vi "Facade.vi"(0 "Data In":T4, 2 "Display State In":T2, 3 "Container State":T3) -> (6 "Data Out":T4, 7 "Display State Out":T2, 8 "Action":T1)   [LabVIEW 2020, in "TTLControlledDevice.xctl"]
uses:
  TTLControlledDevice.xctl
  Data.ctl
  Device Classes/Base Class/TTLControlledDevice.lvclass
  D:/Development/epl-vi-lib/Koop/KObject Class/KObject.lvclass
  <vilib>/_xctls/Container State.ctl
  State.ctl
  <vilib>/_xctls/Action.ctl
  epl-vi-lib/Utility VIs/Controls/KMultilevel Ring/KMultilevel Ring.xctl
  TTLWaterDelivery XControl/TTLWaterDelivery.xctl
  Device Classes/WaterDelivery Class/TTLWaterDelivery.lvclass
  D:/Development/epl-tosca/LV Source/TTL VIs/Device Classes/Base Class/TTLControlledDevice.lvclass
  Device Classes/Base Class/TTLControlledDevice.lvclass/TTLControlledDevice.ctl
  Device Classes/Base Class/Read Line.vi
  Device Classes/Base Class/Read Name.vi
  Device Classes/Base Class/Write Line.vi
  Device Classes/Base Class/Write Name.vi
  <vilib>/DAQmx/write.llb/DAQmx Write (Digital Bool 1Line 1Point).vi
  <vilib>/DAQmx/create/channels.llb/DAQmx Create Channel (DO-Digital Output).vi
  <vilib>/DAQmx/miscellaneous.llb/DAQmx Fill In Error Info.vi
  <vilib>/_xctls/XControlSupport.lvlib
panel:
  in  "Name":string
  out "water cal":bool
  in  "show class":i32
  in  "Class specific":enum32{"Page 1", "Page 2"}(tab)
  in  "Water":refnum<class "TTLWaterDelivery.lvclass">(xcontrol)
  in  "Line":string(xcontrol)
  in  "Test":bool
  out "Icon":picture
  in  "Type":u16(ring)
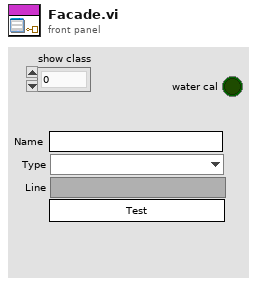
[diagram p1: front panel]
types:
  T1 = typedef "XControlSupport.lvlib/Action.ctl" = cluster{"Data Changed?":bool, "State Changed?":bool, "Action Name":string}
  T2 = typedef "TTLControlledDevice.xctl/State.ctl" = cluster{"Class Map":string[][], "Lines":string[]}
  T3 = typedef "XControlSupport.lvlib/Container State.ctl" = cluster{"Indicator?":bool, "Run Mode?":bool, " Refnum":refnum<vi>}
  T4 = typedef "TTLControlledDevice.xctl/Data.ctl" = refnum<class "TTLControlledDevice.lvclass">
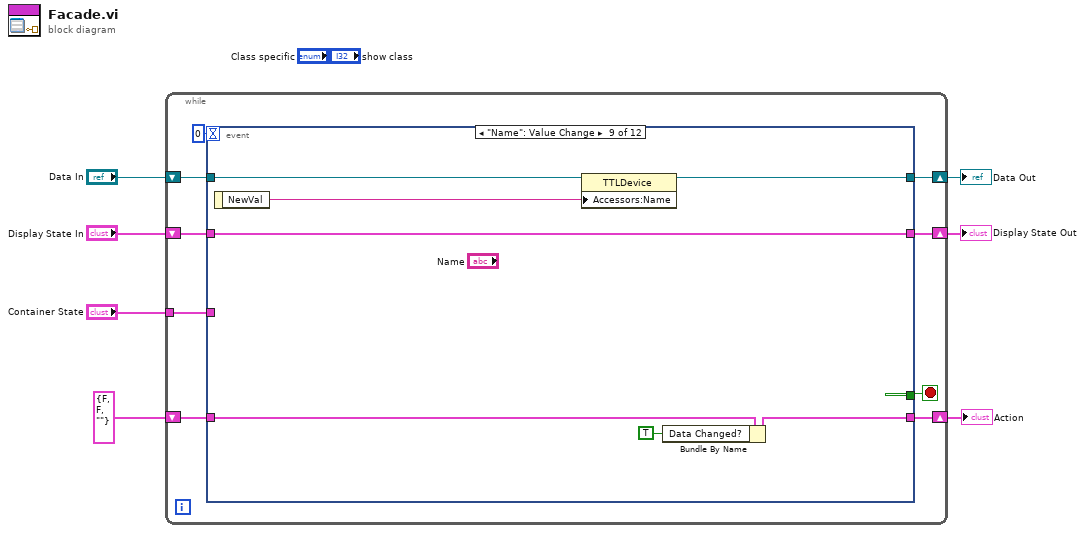
[diagram p0: block diagram]
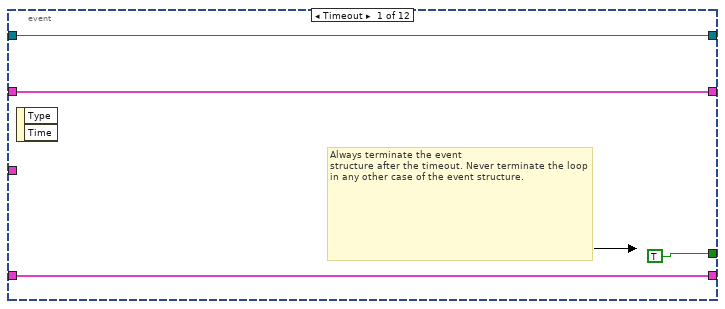
[diagram p2: hidden frame]
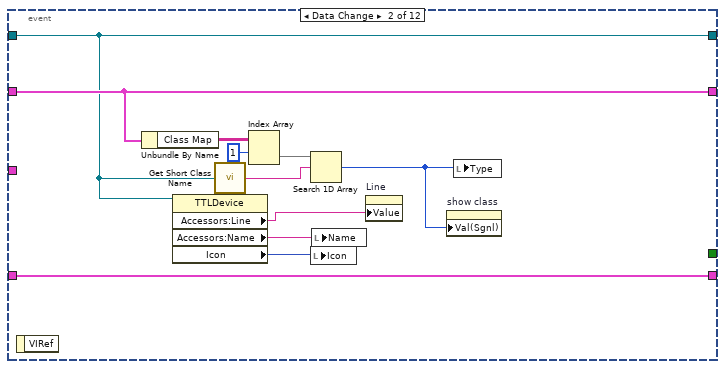
[diagram p3: hidden frame]
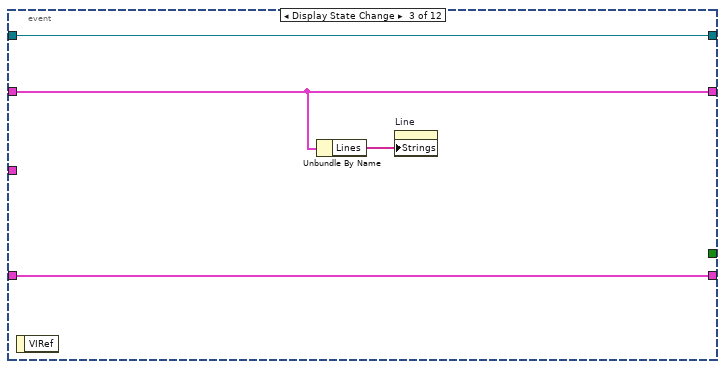
[diagram p4: hidden frame]
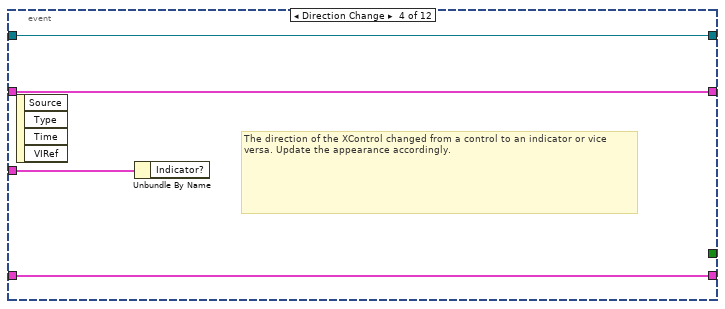
[diagram p5: hidden frame]
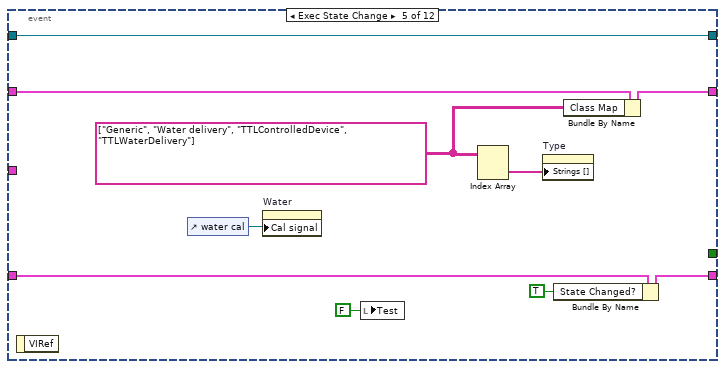
[diagram p6: hidden frame]
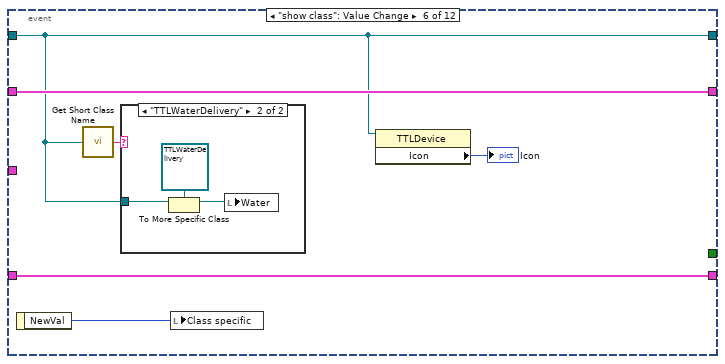
[diagram p7: hidden frame]
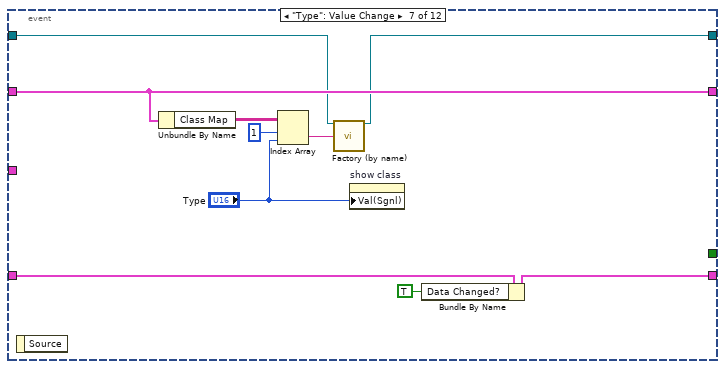
[diagram p9: hidden frame]
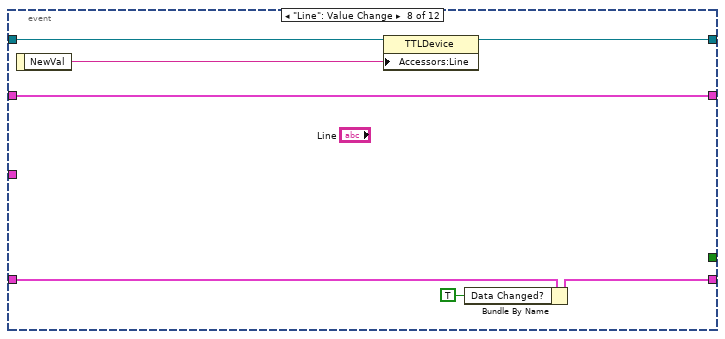
[diagram p10: hidden frame]
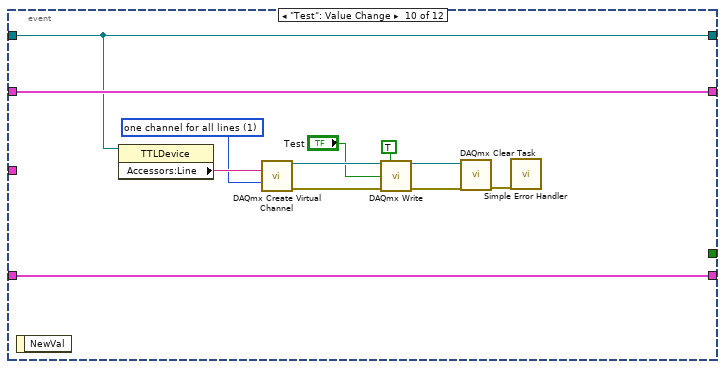
[diagram p11: hidden frame]
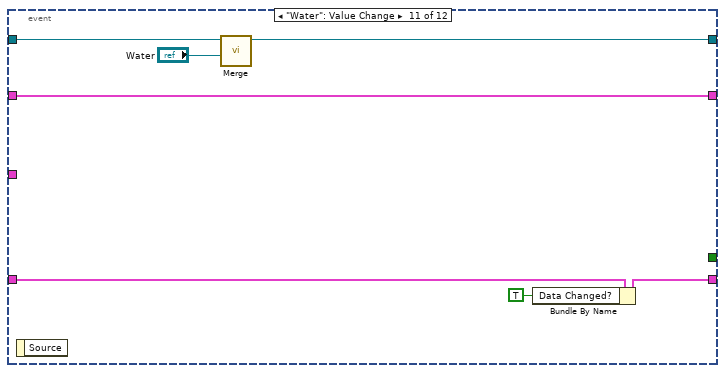
[diagram p12: hidden frame]
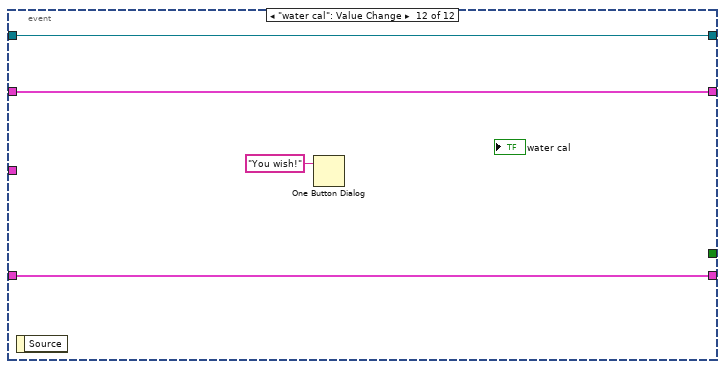
[diagram p13: hidden frame]
diagram:
  n1 = while {
    shift-right: [w15] -> w4
    shift-left: "Display State In" -> [w16]
    tunnel: "Container State" -> [w12]
    shift-right: [w10] -> w7
    shift-left: "Data In" -> [w11]
    shift-right: [w8] -> w2
    shift-left: T1 {"Data Changed?"=FALSE, "State Changed?"=FALSE, "Action Name"=""} ("Action") -> [w9]
    stop <- w14 stop-if-true
    n2 = event shown="[8] \"Name\": Value Change" {
      selector: _ -> [_ _ _ _ _ _ _ _ _ _ _ _]
      dyn-events: _ -> [_ _ _ _ _ _ _ _ _ _ _ _]
      timeout: 0 -> [_ _ _ _ _ _ _ _ _ _ _ _]
      tunnel: w16 -> [w18 w30 w33 w38 w49 w55 w67 w75 w82 w94 w101 w105]
      tunnel: [w18 w30 w33 w38 w46 w55 w67 w75 w82 w94 w101 w105] -> w15
      tunnel: [TRUE _ _ _ _ _ _ _ _ _ _ _] -> w14
      tunnel: w12 -> [_ _ _ w39 _ _ _ _ _ _ _ _]
      tunnel: w11 -> [w17 w27 w35 w37 w48 w51 w61 w74 w81 w92 w99 w104]
      tunnel: [w17 w27 w35 w37 w48 w51 w59 w70 w77 w92 w98 w104] -> w10
      tunnel: [w19 w31 w34 w36 w45 w54 w63 w72 w79 w93 w96 w103] -> w8
      tunnel: w9 -> [w19 w31 w34 w36 w47 w54 w68 w73 w80 w93 w100 w103]
      event Timeout {
        # "Always terminate the event\nstructure after the timeout. Never terminate the loop in any other case of the event structure."
        n3 = event-data() -> ()  [unwired: 1 in, 2 out]
      }
      event Data Change {
        n4 = event-data() -> ()  [unwired: 1 in, 1 out]
        n5 = Unbundle By Name(w30) -> ("Class Map"=w29:string[][])
        n6 = property class="TTLDevice"(reference=w27) -> ("Accessors:Line"=w24:string, "Accessors:Name"=w21:string, "Icon"=w22:picture)  [unwired: 1 in, 2 out]
        n7 = call "Get Short Class Name.vi"("KObject in"=w27) -> ("Class"=w25:string)  [unwired: 4 in]
        n8 = Index Array(array=w29, index (row)=1) -> (element=w26:string[])  [unwired: 1 in]
        n9 = Search 1D Array(1D array=w26, element=w25) -> (index of element=w23:i32)  [unwired: 1 in]
        n10 = local write "Icon"(w22) -> ()
        n11 = local write "Name"(w21) -> ()
        n12 = property on="Line" class="KMultilevel Ring (strict)"("Value"=w24) -> ()  [unwired: 2 in, 2 out]
        n13 = property on="show class" class="DigNum (strict)"("Val(Sgnl)"=w23) -> ()  [unwired: 2 in, 2 out]
        n14 = local write "Type"(w23) -> ()
      }
      event Display State Change {
        n15 = event-data() -> ()  [unwired: 1 in, 1 out]
        n16 = Unbundle By Name(w33) -> ("Lines"=w32:string[])
        n17 = property on="Line" class="KMultilevel Ring (strict)"("Strings"=w32) -> ()  [unwired: 2 in, 2 out]
      }
      event Direction Change {
        # "The direction of the XControl changed from a control to an indicator or vice versa. Update the appearance accordingly."
        n18 = event-data() -> ()  [unwired: 1 in, 4 out]
        n19 = Unbundle By Name(w39) -> ()  [unwired: 1 out]
      }
      event Exec State Change {
        w43 = string[][] [["Generic", "Water delivery"], ["TTLControlledDevice", "TTLWaterDelivery"]]
        n20 = event-data() -> ()  [unwired: 1 in, 1 out]
        n21 = control-ref of="water cal"() -> (w40:refnum<vi>)
        n22 = property on="Water" class="TTLWaterDelivery (strict)"("Cal signal"=w40) -> ()  [unwired: 2 in, 2 out]
        n23 = local write "Test"(FALSE ("Test")) -> ()
        n24 = Index Array(array=w43) -> (element=w42:string[])  [unwired: 2 in]
        n25 = property on="Type" class="Ring (strict)"("Strings []"=w42) -> ()  [unwired: 2 in, 2 out]
        n26 = Bundle By Name(cluster=w47, "State Changed?"=TRUE) -> (w45:T1)
        n27 = Bundle By Name(cluster=w49, "Class Map"=w43) -> (w46:T2)
      }
      event "show class": Value Change {
        n28 = event-data() -> ("NewVal"=w52:i32)  [unwired: 1 in]
        n29 = call "Get Short Class Name.vi"("KObject in"=w51) -> ("Class"=w50:string)  [unwired: 4 in]
        n30 = case shown="\"TTLWaterDelivery\"" w50 {
          tunnel: w51 -> [_ w58]
          frame "TTLControlledDevice", Default {
          }
          frame "TTLWaterDelivery" {
            n31 = To More Specific Class(target class=refnum<class "TTLWaterDelivery.lvclass"> refnum ("TTLWater"), reference=w58) -> (specific class reference=w57:refnum<class "TTLWaterDelivery.lvclass">)  [unwired: 1 in, 1 out]
            n32 = local write "Water"(w57) -> ()
          }
        }
        n33 = local write "Class specific"(w52) -> ()
        n34 = property class="TTLDevice"(reference=w51) -> ("Icon"=→"Icon":picture)  [unwired: 1 in, 2 out]
      }
      event "Type": Value Change {
        n35 = event-data() -> ()  [unwired: 1 in, 1 out]
        n36 = Unbundle By Name(w67) -> ("Class Map"=w66:string[][])
        n37 = Index Array(array=w66, index (row)=1 ("disabled index (row)"), index (col)="Type") -> (element=w64:string)
        n38 = call "Factory (by name).vi"("TTLDevice in"=w61, "Class Name"=w64) -> ("TTLDevice out"=w59:refnum<class "TTLControlledDevice.lvclass">)  [unwired: 12 in, 1 out]
        n39 = property on="show class" class="DigNum (strict)"("Val(Sgnl)"="Type") -> ()  [unwired: 2 in, 2 out]
        n40 = Bundle By Name(cluster=w68, "Data Changed?"=TRUE) -> (w63:T1)
      }
      event "Line": Value Change {
        n41 = event-data() -> ("NewVal"=w69:string)  [unwired: 1 in]
        n42 = property class="TTLDevice"(reference=w74, "Accessors:Line"=w69) -> (reference out=w70:T4)  [unwired: 1 in, 1 out]
        n43 = Bundle By Name(cluster=w73, "Data Changed?"=TRUE) -> (w72:T1)
      }
      event "Name": Value Change {
        n44 = event-data() -> ("NewVal"=w76:string)  [unwired: 1 in]
        n45 = property class="TTLDevice"(reference=w81, "Accessors:Name"=w76) -> (reference out=w77:T4)  [unwired: 1 in, 1 out]
        n46 = Bundle By Name(cluster=w80, "Data Changed?"=TRUE) -> (w79:T1)
      }
      event "Test": Value Change {
        w90 = 1 items=["one channel for each line", "one channel for all lines"] ("line grouping")
        n47 = event-data() -> ()  [unwired: 1 in, 1 out]
        n48 = property class="TTLDevice"(reference=w92) -> ("Accessors:Line"=w91:string)  [unwired: 1 in, 2 out]
        n49 = call-poly <vilib>:"DAQmx Create Virtual Channel.vi"("lines"=w91, "line grouping"=w90) -> ("task out"=w89:refnum<k21>, "error out"=w88:errorcluster)  [unwired: 12 in]
        n50 = call-poly <vilib>:"DAQmx Write.vi"("task/channels in"=w89, "auto start"=TRUE, "data"="Test", "error in"=w88) -> ("task out"=w86:refnum<k21>, "error out"=w85:errorcluster)  [unwired: 9 in, 1 out]
        n51 = call <vilib>:"DAQmx Clear Task.vi"("task in"=w86, "error in"=w85) -> ("error out"=w84:errorcluster)  [unwired: 13 in]
        n52 = call <vilib>:"Simple Error Handler.vi"("error in (no error)"=w84) -> ()  [unwired: 4 in, 5 out]
      }
      event "Water": Value Change {
        n53 = event-data() -> ()  [unwired: 1 in, 1 out]
        n54 = call "Merge.vi"("TTLDevice in 2"="Water", "TTLDevice in"=w99) -> ("TTLDevice out"=w98:T4)  [unwired: 8 in, 1 out]
        n55 = Bundle By Name(cluster=w100, "Data Changed?"=TRUE) -> (w96:T1)
      }
      event "water cal": Value Change {
        n56 = event-data() -> ()  [unwired: 1 in, 1 out]
        n57 = One Button Dialog(message="You wish!") -> ()  [unwired: 1 in, 1 out]
      }
    }
  }
  "Display State Out" <- w4
  "Data Out" <- w7
  "Action" <- w2
